vi "passTestNew.vi"(10 "Initial channel":T2) -> (0 "Enum 2":T1)   [LabVIEW 2017]
uses:
  passTestStates.ctl
  <extravilib>/ChannelInstances/Lossy Stream-t'AI Input.ctl'/)Channel.ctl
  Core/AI Input.ctl
  Core/AI Robot.ctl
  Intel/Functions Enum.ctl
  Intel/AttackerStates.ctl
  Core/AI Ball.ctl
  Core/Field Size.ctl
  Core/AI Judge.ctl
  Intel/Command Enum.ctl
  Util/Events/Events.ctl
  <extravilib>/ChannelInstances/Lossy Stream-dbl/Read With Abort.vi
  <extravilib>/ChannelInstances/Lossy Stream-t'AI Input.ctl'/Read With Abort.vi
  <extravilib>/ChannelInstances/Lossy Stream-t'passTestStates.ctl'/Write With Abort.vi
  <extravilib>/ChannelInstances/Lossy Stream-t'passTestStates.ctl'/Read With Abort.vi
  <extravilib>/ChannelInstances/Lossy Stream-dbl/Write With Abort.vi
  <extravilib>/ChannelInstances/Lossy Stream-t'AI Input.ctl'/Write With Abort.vi
  <extravilib>/ChannelInstances/Lossy Stream-dbl/EndpointRead.vi
  <extravilib>/ChannelInstances/Lossy Stream-t'AI Input.ctl'/EndpointRead.vi
  <extravilib>/ChannelInstances/Lossy Stream-t'passTestStates.ctl'/Endpoint.vi
  <extravilib>/ChannelInstances/Lossy Stream-t'passTestStates.ctl'/EndpointRead.vi
  <extravilib>/ChannelInstances/Lossy Stream-dbl/Endpoint.vi
  <extravilib>/ChannelInstances/Lossy Stream-t'AI Input.ctl'/Endpoint.vi
  <extravilib>/ChannelInstances/Lossy Stream-t'AI Input.ctl'/Instantiate.vi
  <extravilib>/ChannelInstances/Lossy Stream-t'AI Input.ctl'/)Channel.vi
  <resource>/ChannelSupport/_ChannelSupport/WaitIfNeeded.vi
  <extravilib>/ChannelInstances/Lossy Stream-t'passTestStates.ctl'/Instantiate.vi
  <extravilib>/ChannelInstances/Lossy Stream-t'passTestStates.ctl'/)Channel.vi
  <extravilib>/ChannelInstances/Lossy Stream-dbl/Instantiate.vi
  <extravilib>/ChannelInstances/Lossy Stream-dbl/)Channel.vi
  <extravilib>/ChannelInstances/Lossy Stream-t'passTestStates.ctl'.lvlib
  <extravilib>/ChannelInstances/Lossy Stream-t'AI Input.ctl'.lvlib
  <extravilib>/ChannelInstances/Lossy Stream-dbl.lvlib
panel:
  out "Enum":T1
  out "ID Kicker Robot":dbl
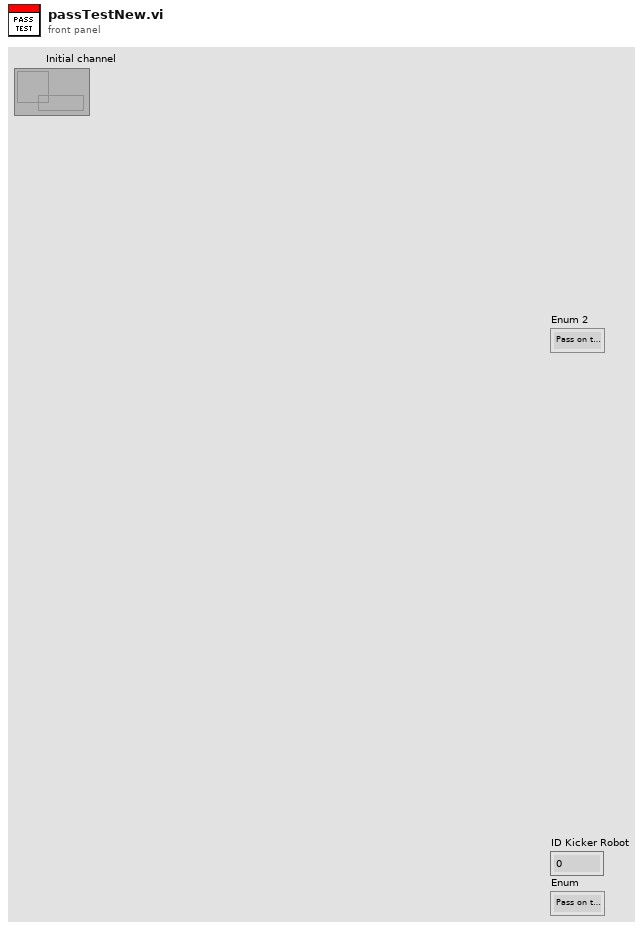
[diagram p1: front panel]
types:
  T1 = typedef "passTestStates.ctl" = enum16{"Pass on the way", "Ball stops", "Pass intercepted", "Ball out of the field", "Ball missed robot", "Need more force to pass", "Too much force", "Correct pass", "Keep ball possesion", "Robot kicked the ball"}
  T2 = typedef "Lossy Stream-t'AI Input.ctl'.lvlib/)Channel.ctl" = refnum<queue>
  T3 = typedef "AI Input.ctl" = cluster{"our_robots":T4[], "enemy_robots":T4[], "balls":T7[], "geometry":T8, "IA Judge":T9, "Received Timestamp":timestamp, "Events":T11}
  T4 = typedef "AI Robot.ctl" = cluster{"id":u32, "function":T5, "x":dbl, "y":dbl, "orientation":dbl, "v_tangent":dbl, "v_normal":dbl, "v_ang":dbl, "kick_x":dbl, "kick_z":dbl, "dribble":bool, "Timestamp":timestamp, "dest_x":dbl, "dest_y":dbl, "dest_orientation":dbl, "estimatives":cluster{"est_v_tangent":dbl, "est_v_normal":dbl, "est_vx":dbl, "est_vy":dbl, "Pos Robot Est":dbl[]}, "dest_x_kick":dbl, "dest_y_kick":dbl, "Gap Coord":dbl[], "States":T6}
  T5 = typedef "Functions Enum.ctl" = enum16{"Attacker", "Goalie", "Defender", "Striker", "Goto 0", "Dummy", "Kicker", "ZigZag"}
  T6 = typedef "AttackerStates.ctl" = enum16{"Pass", "GoToTangent", "BallGetting", "GoToKick", ""}
  T7 = typedef "AI Ball.ctl" = cluster{"x":dbl, "y":dbl, "timestamp":timestamp, "Vel_x":dbl, "Vel_y":dbl, "Pos Bola Est":dbl[]}
  T8 = typedef "Field Size.ctl" = cluster{"line_width":u32, "field_length":u32, "field_width":u32, "boundary_width":u32, "referee_width":u32, "goal_width":u32, "goal_depth":u32, "goal_wall_width":u32, "center_circle_radius":u32, "defense_radius":u32, "defense_stretch":u32, "free_kick_from_defense_dist":u32, "penalty_spot_from_field_line_dist":u32, "penalty_line_from_spot_dist":u32}
  T9 = typedef "AI Judge.ctl" = cluster{"stage":string, "command":string, "our_goalie_id":dbl, "enemy_goalie_id":dbl, "command enum":T10, "Time":enum16{"Azul", "Amarelo"}}
  T10 = typedef "Command Enum.ctl" = enum16{"Halt", "Stop", "Force Start", "PKA Normal Start", "Prepare Kickoff Ally", "PKE Normal Start", "Prepare Kickoff Enemy", "Prepare Penalty Ally", "PPA Normal Start", "Prepare Penalty Enemy", "PPE Normal Start", "Direct Free Enemy", "Direct Free Ally", "Indirect Free Enemy", "Indirect Free Ally", "Timeout Enemy", "Timeout Ally", "Goal Enemy", "Goal Ally", "Ball Placement Enemy", "Ball Placement Ally", "Normal Half Time", "Extra Time Break", "Extra Half Time", "None", "Post Game"}
  T11 = typedef "Events.ctl" = cluster{"Touch":bool, "Ball out":bool, "id touch":dbl, "Ball out of \nVision":bool, "Ball inside \nGoalie area":bool, "Robot not responding":bool, "Robots responding status":dbl[], "Enemy Ball \nPossession":bool, "Pass State":bool, "id end of pass":dbl, "Kick":bool, "Id ini Possession":dbl, "Ball Possesion":bool, "Id Possesion":dbl}
  T12 = typedef "Lossy Stream-t'passTestStates.ctl'.lvlib/)Channel.ctl" = refnum<queue>
  T13 = typedef "Lossy Stream-dbl.lvlib/)Channel.ctl" = refnum<queue>
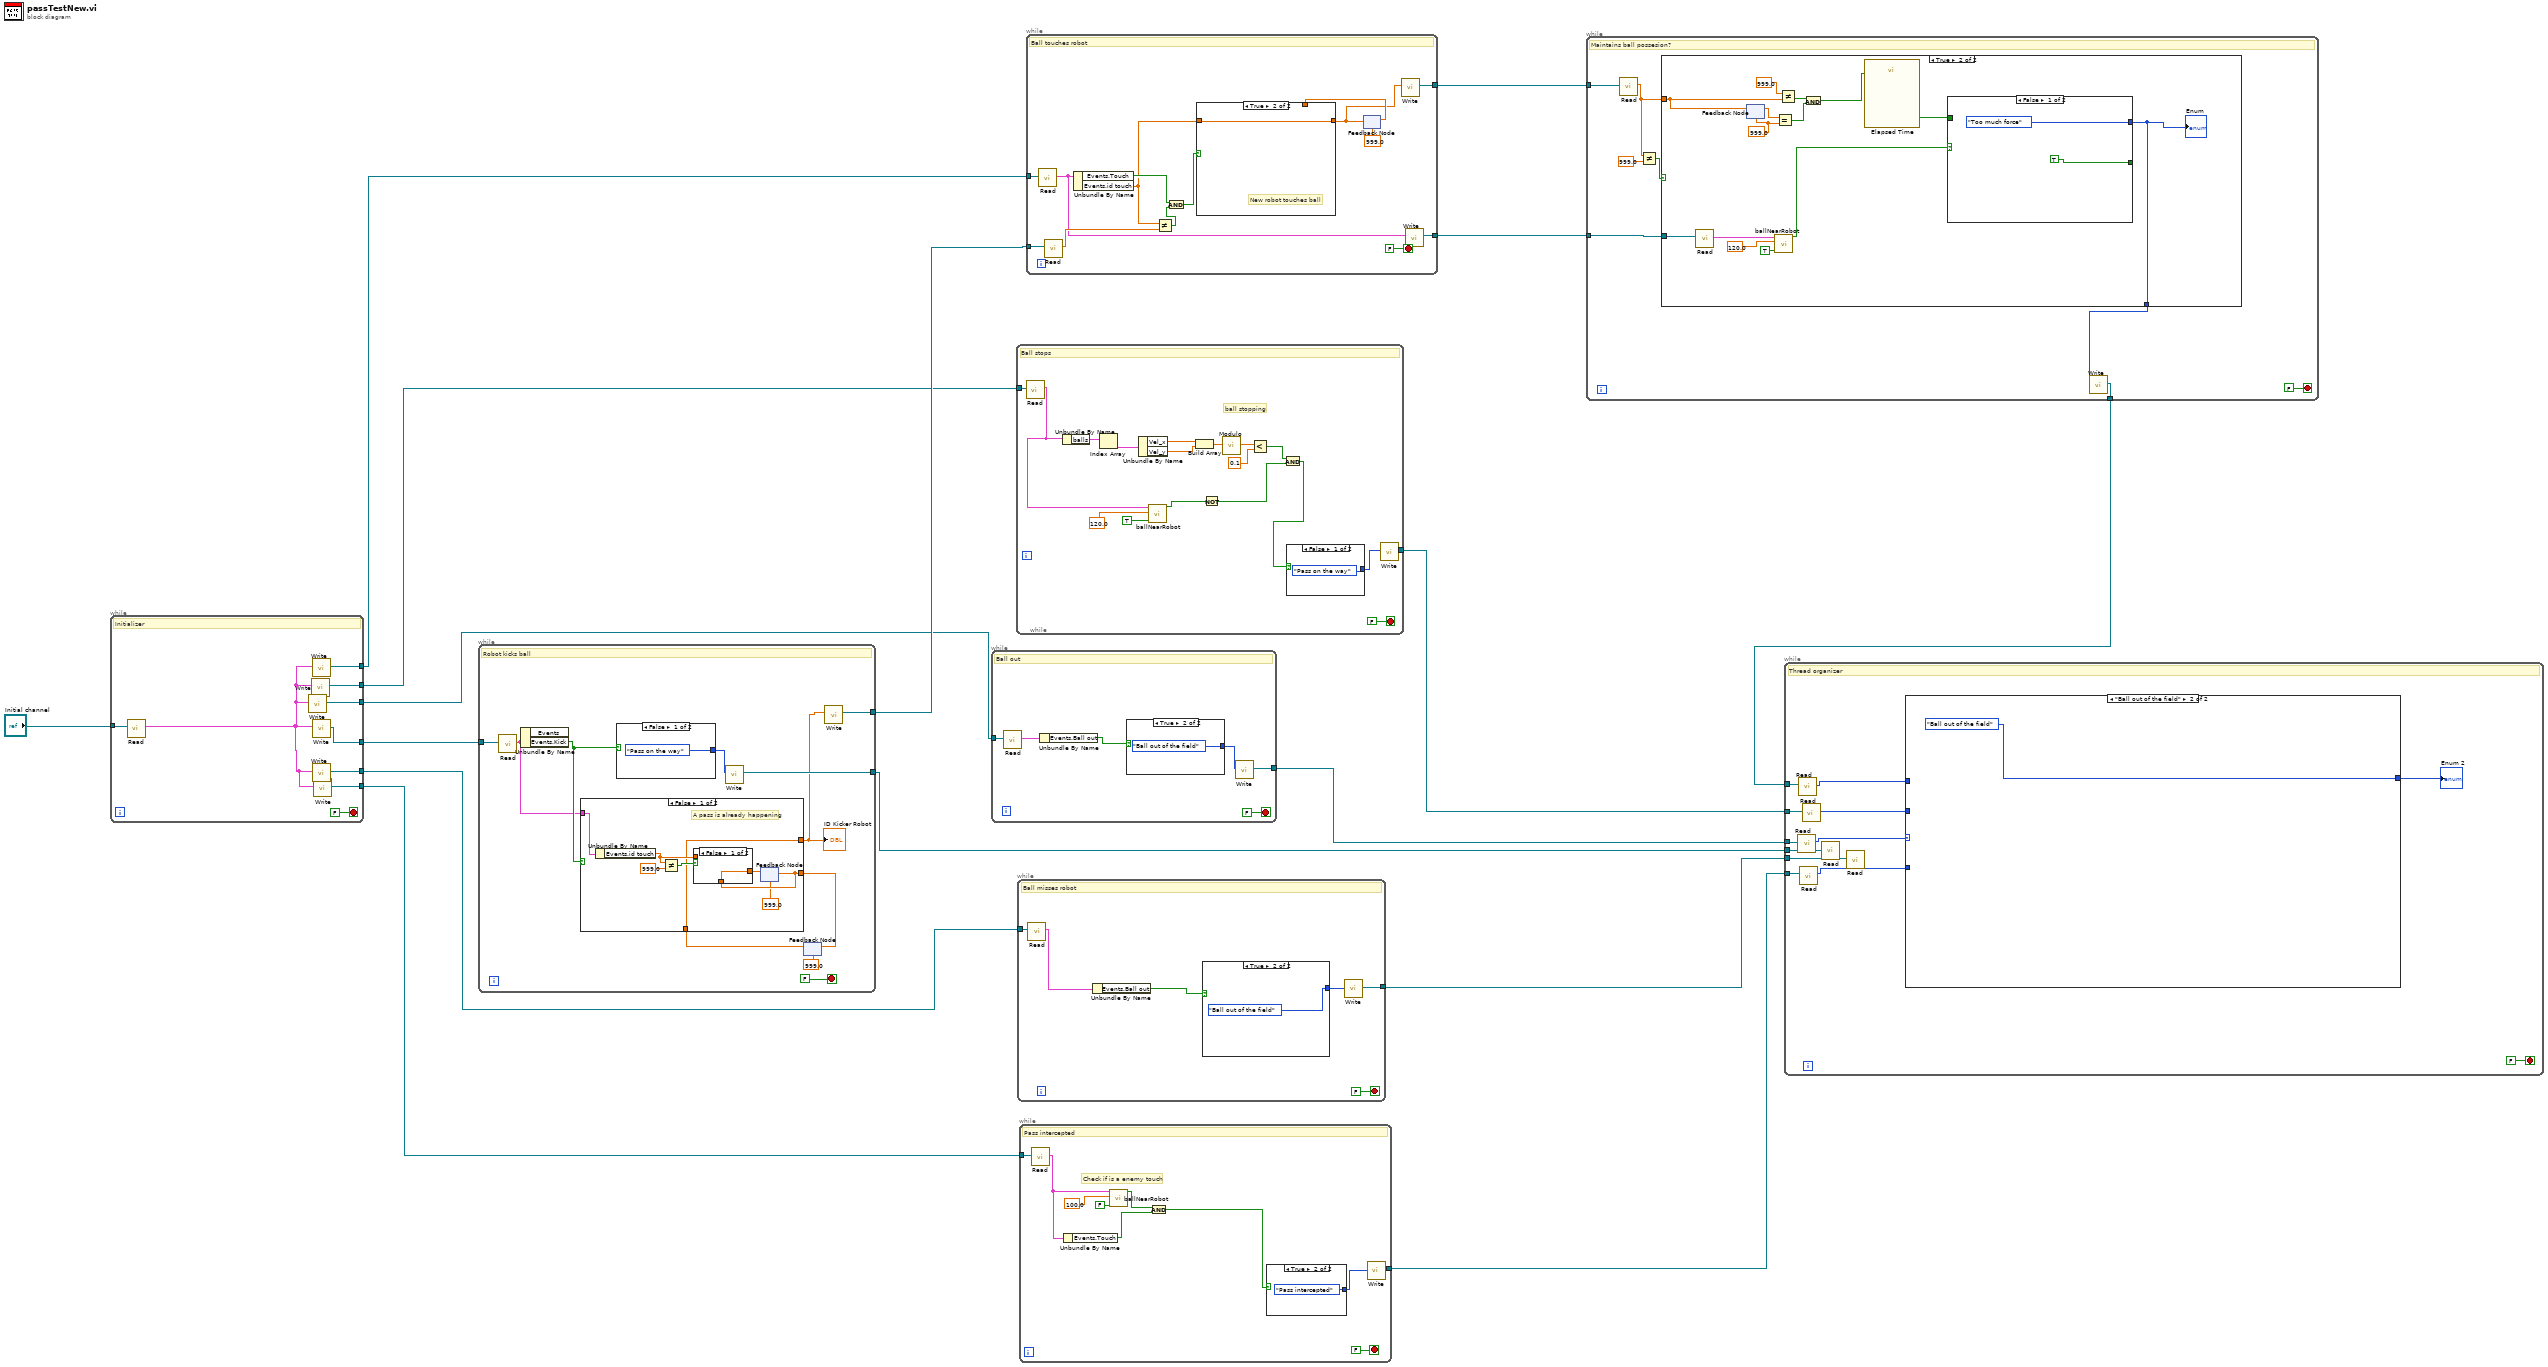
[diagram p0: block diagram]
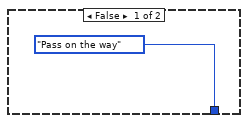
[diagram p2: hidden frame]
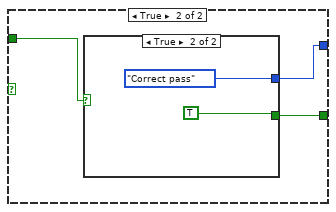
[diagram p3: hidden frame]
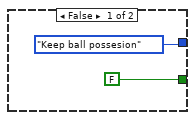
[diagram p4: hidden frame]
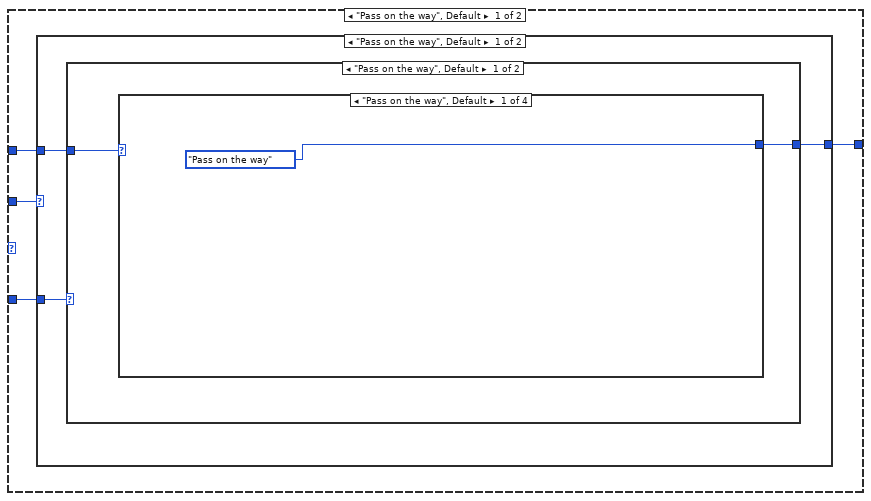
[diagram p5: hidden frame]
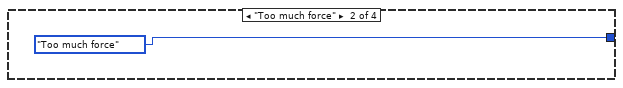
[diagram p6: hidden frame]
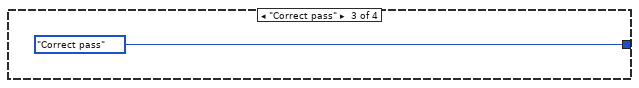
[diagram p7: hidden frame]
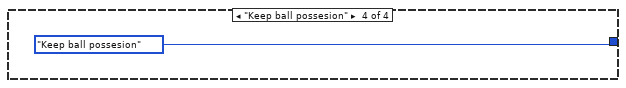
[diagram p8: hidden frame]
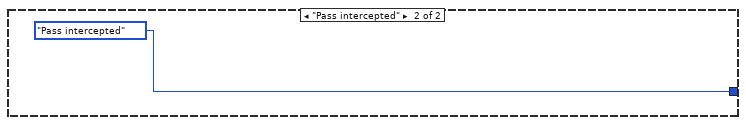
[diagram p9: hidden frame]
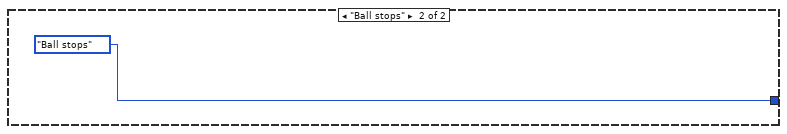
[diagram p10: hidden frame]
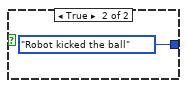
[diagram p14: hidden frame]
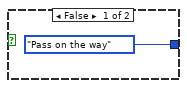
[diagram p15: hidden frame]
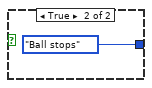
[diagram p16: hidden frame]
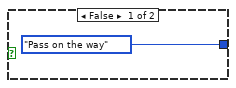
[diagram p17: hidden frame]
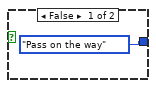
[diagram p18: hidden frame]
diagram:
  n1 = while {
    tunnel: "Initial channel" -> [w25]
    tunnel: [w24] -> w6
    tunnel: [w23] -> w3
    tunnel: [w21] -> w5
    tunnel: [w20] -> w4
    tunnel: [w19] -> w2
    tunnel: [w17] -> w1
    stop <- FALSE stop-if-true
    # "Initializer"
    n2 = call <extravilib>:"Read.vi"("channel"=w25) -> ("element"=w18:T3)  [unwired: 5 in, 5 out]
    n3 = call <extravilib>:"Write.vi"("element"=w18) -> ("channel"=w23:T2)  [unwired: 8 in, 2 out]
    n4 = call <extravilib>:"Write.vi"("element"=w18) -> ("channel"=w19:T2)  [unwired: 8 in, 2 out]
    n5 = call <extravilib>:"Write.vi"("element"=w18) -> ("channel"=w17:T2)  [unwired: 8 in, 2 out]
    n6 = call <extravilib>:"Write.vi"("element"=w18) -> ("channel"=w24:T2)  [unwired: 8 in, 2 out]
    n7 = call <extravilib>:"Write.vi"("element"=w18) -> ("channel"=w20:T2)  [unwired: 8 in, 2 out]
    n8 = call <extravilib>:"Write.vi"("element"=w18) -> ("channel"=w21:T2)  [unwired: 8 in, 2 out]
  }
  n9 = while {
    tunnel: [w35] -> w8
    tunnel: w6 -> [w33]
    tunnel: [w27] -> w16
    stop <- FALSE stop-if-true
    # "Robot kicks ball"
    n10 = call <extravilib>:"Read.vi"("channel"=w33) -> ("element"=w31:T3)  [unwired: 5 in, 5 out]
    n11 = Unbundle By Name(w31) -> ("Events.Kick"=w32:bool)  [unwired: 1 out]
    n12 = case shown="False" w32 {
      tunnel: [passTestStates."Pass on the way" passTestStates."Robot kicked the ball"] -> w34
      frame False {
      }
      frame True {
      }
    }
    n13 = call <extravilib>:"Write.vi"("element"=w34) -> ("channel"=w35:T12)  [unwired: 8 in, 2 out]
    n14 = feedback #1(999.0 ("id touch")) -> (w29:dbl)
    n15 = case shown="False" w32 {
      tunnel: w31 -> [w44 _]
      tunnel: [w39 w47] -> w30
      tunnel: w29 -> [w37 w47]
      tunnel: [w37 w47] -> w28
      frame False {
        # "A pass is already happening"
        n16 = Unbundle By Name(w44) -> ("Events.id touch"=w41:dbl)
        n17 = Not Equal?(x=w41, y=999.0) -> (x != y?=w42:bool)
        n18 = feedback #2(999.0 ("id touch")) -> (w39:dbl)
        n19 = case shown="False" w42 {
          tunnel: w41 -> [_ w46]
          tunnel: [w45 w46] -> w40
          tunnel: w39 -> [w45 _]
          frame False {
          }
          frame True {
          }
        }
        n20 = feedback-in #2(w40) -> ()
      }
      frame True {
        # "A new pass is starting"
      }
    }
    "ID Kicker Robot" <- w28
    n21 = feedback-in #1(w30) -> ()
    n22 = call <extravilib>:"Write.vi"("element"=w28) -> ("channel"=w27:T13)  [unwired: 8 in, 2 out]
  }
  n23 = while {
    tunnel: [w54] -> w11
    tunnel: w3 -> [w51]
    stop <- FALSE stop-if-true
    # "Ball out"
    n24 = call <extravilib>:"Read.vi"("channel"=w51) -> ("element"=w50:T3)  [unwired: 5 in, 5 out]
    n25 = Unbundle By Name(w50) -> ("Events.Ball out"=w53:bool)
    n26 = case shown="True" w53 {
      tunnel: [passTestStates."Pass on the way" passTestStates."Ball out of the field"] -> w52
      frame False {
      }
      frame True {
      }
    }
    n27 = call <extravilib>:"Write.vi"("element"=w52) -> ("channel"=w54:T12)  [unwired: 8 in, 2 out]
  }
  n28 = while {
    tunnel: w2 -> [w60]
    tunnel: [w58] -> w10
    stop <- FALSE stop-if-true
    # "ball stopping"
    # "Ball stops"
    n29 = call <extravilib>:"Read.vi"("channel"=w60) -> ("element"=w59:T3)  [unwired: 5 in, 5 out]
    n30 = Unbundle By Name(w59) -> ("balls"=w75:T7[])
    n31 = Index Array(array=w75) -> (element=w74:T7)  [unwired: 1 in]
    n32 = Unbundle By Name(w74) -> ("Vel_x"=w73:dbl, "Vel_y"=w72:dbl)
    n33 = call "ballNearRobot.vi"("Our robots?"=TRUE, "Distance"=120.0, "IA state"=w59) -> ("Near to some robot"=w67:bool)  [unwired: 7 in, 1 out]
    n34 = Build Array(w73, w72) -> (w71:dbl[])
    n35 = Not(x=w67) -> (.not. x?=w64:bool)
    n36 = call "Modulo.vi"("2D vector"=w71) -> ("Modulo"=w70:dbl)  [unwired: 10 in]
    n37 = Less?(x=w70, y=0.1) -> (x < y?=w68:bool)
    n38 = And(x=w68, y=w64) -> (x .and. y?=w61:bool)
    n39 = case shown="False" w61 {
      tunnel: [passTestStates."Pass on the way" passTestStates."Ball stops"] -> w62
      frame False {
      }
      frame True {
      }
    }
    n40 = call <extravilib>:"Write.vi"("element"=w62) -> ("channel"=w58:T12)  [unwired: 8 in, 2 out]
  }
  n41 = while {
    tunnel: [w81] -> w12
    tunnel: w4 -> [w80]
    stop <- FALSE stop-if-true
    # "Ball misses robot"
    n42 = call <extravilib>:"Read.vi"("channel"=w80) -> ("element"=w79:T3)  [unwired: 5 in, 5 out]
    n43 = Unbundle By Name(w79) -> ("Events.Ball out"=w78:bool)
    n44 = case shown="True" w78 {
      tunnel: [passTestStates."Pass on the way" passTestStates."Ball out of the field"] -> w82
      frame False {
      }
      frame True {
      }
    }
    n45 = call <extravilib>:"Write.vi"("element"=w82) -> ("channel"=w81:T12)  [unwired: 8 in, 2 out]
  }
  n46 = while {
    tunnel: w5 -> [w91]
    tunnel: [w86] -> w13
    stop <- FALSE stop-if-true
    # "Check if is a enemy touch"
    # "Pass intercepted"
    n47 = call <extravilib>:"Read.vi"("channel"=w91) -> ("element"=w90:T3)  [unwired: 5 in, 5 out]
    n48 = Unbundle By Name(w90) -> ("Events.Touch"=w89:bool)
    n49 = call "ballNearRobot.vi"("Our robots?"=FALSE, "Distance"=100.0, "IA state"=w90) -> ("Near to some robot"=w93:bool)  [unwired: 7 in, 1 out]
    n50 = And(x=w93, y=w89) -> (x .and. y?=w88:bool)
    n51 = case shown="True" w88 {
      tunnel: [passTestStates."Pass on the way" passTestStates."Pass intercepted"] -> w87
      frame False {
      }
      frame True {
      }
    }
    n52 = call <extravilib>:"Write.vi"("element"=w87) -> ("channel"=w86:T12)  [unwired: 8 in, 2 out]
  }
  n53 = while {
    tunnel: w1 -> [w110]
    tunnel: w16 -> [w108]
    tunnel: [w100] -> w15
    tunnel: [w98] -> w14
    stop <- FALSE stop-if-true
    # "Ball touches robot"
    n54 = call <extravilib>:"Read.vi"("channel"=w110) -> ("element"=w99:T3)  [unwired: 5 in, 5 out]
    n55 = call <extravilib>:"Read.vi"("channel"=w108) -> ("element"=w107:dbl)  [unwired: 5 in, 5 out]
    n56 = Unbundle By Name(w99) -> ("Events.Touch"=w106:bool, "Events.id touch"=w103:dbl)
    n57 = Not Equal?(x=w103, y=w107) -> (x != y?=w105:bool)
    n58 = And(x=w106, y=w105) -> (x .and. y?=w104:bool)
    n59 = feedback #3(999.0 ("id touch")) -> (w102:dbl)
    n60 = case shown="True" w104 {
      tunnel: w103 -> [_ w113]
      tunnel: [w112 w113] -> w101
      tunnel: w102 -> [w112 _]
      frame False {
      }
      frame True {
        # "New robot touches ball"
      }
    }
    n61 = feedback-in #3(w101) -> ()
    n62 = call <extravilib>:"Write.vi"("element"=w101) -> ("channel"=w100:T13)  [unwired: 8 in, 2 out]
    n63 = call <extravilib>:"Write.vi"("element"=w99) -> ("channel"=w98:T2)  [unwired: 8 in, 2 out]
  }
  n64 = while {
    tunnel: w15 -> [w117]
    tunnel: w14 -> [w120]
    tunnel: [w118] -> w9
    stop <- FALSE stop-if-true
    # "Maintains ball possesion?"
    n65 = call <extravilib>:"Read.vi"("channel"=w117) -> ("element"=w115:dbl)  [unwired: 5 in, 5 out]
    n66 = Not Equal?(x=w115, y=999.0) -> (x != y?=w114:bool)
    n67 = case shown="True" w114 {
      tunnel: w120 -> [_ w134]
      tunnel: [passTestStates."Pass on the way" w124] -> w119
      tunnel: w115 -> [_ w123]
      frame False {
      }
      frame True {
        w131 = 999.0 ("element")
        n68 = call <extravilib>:"Read.vi"("channel"=w134) -> ("element"=w133:T3)  [unwired: 5 in, 5 out]
        n69 = feedback #4(w131) -> (w130:dbl)
        n70 = feedback-in #4(w123) -> ()
        n71 = call "ballNearRobot.vi"("Our robots?"=TRUE, "Distance"=120.0, "IA state"=w133) -> ("Near to some robot"=w132:bool)  [unwired: 7 in, 1 out]
        n72 = Equal?(x=w130, y=w131) -> (x = y?=w129:bool)
        n73 = Not Equal?(x=999.0 ("element"), y=w123) -> (x != y?=w128:bool)
        n74 = And(x=w128, y=w129) -> (x .and. y?=w126:bool)
        n75 = call "Elapsed Time"("Reset"=w126) -> ("Time has Elapsed"=w125:bool)  [unwired: 11 in, 7 out]
        n76 = case shown="False" w132 {
          tunnel: [passTestStates."Too much force" w141] -> w124
          tunnel: [TRUE ("y") w140] -> _
          tunnel: w125 -> [_ w139]
          frame False {
          }
          frame True {
            n77 = case shown="True" w139 {
              tunnel: [passTestStates."Keep ball possesion" passTestStates."Correct pass"] -> w141
              tunnel: [FALSE ("y") TRUE ("y")] -> w140
              frame False {
              }
              frame True {
              }
            }
          }
        }
        "Enum" <- w124
      }
    }
    n78 = call <extravilib>:"Write.vi"("element"=w119) -> ("channel"=w118:T12)  [unwired: 8 in, 2 out]
  }
  n79 = while {
    tunnel: w13 -> [w151]
    tunnel: w12 -> [w152]
    tunnel: w11 -> [w154]
    tunnel: w10 -> [w155]
    tunnel: w9 -> [w156]
    tunnel: w8 -> [w153]
    stop <- FALSE stop-if-true
    # "Thread organizer"
    n80 = call <extravilib>:"Read.vi"("channel"=w154) -> ("element"=w150:T1)  [unwired: 5 in, 5 out]
    n81 = call <extravilib>:"Read.vi"("channel"=w156) -> ("element"=w147:T1)  [unwired: 5 in, 5 out]
    n82 = call <extravilib>:"Read.vi"("channel"=w151) -> ("element"=w148:T1)  [unwired: 5 in, 5 out]
    n83 = call <extravilib>:"Read.vi"("channel"=w155) -> ("element"=w149:T1)  [unwired: 5 in, 5 out]
    n84 = call <extravilib>:"Read.vi"("channel"=w153) -> ()  [unwired: 5 in, 6 out]
    n85 = call <extravilib>:"Read.vi"("channel"=w152) -> ()  [unwired: 5 in, 6 out]
    n86 = case shown="\"Ball out of the field\"" w150 {
      tunnel: w149 -> [w161 _]
      tunnel: w148 -> [w160 _]
      tunnel: w147 -> [w159 _]
      tunnel: [w158 passTestStates."Ball out of the field"] -> w146
      frame "Pass on the way", Default {
        n87 = case shown="\"Pass on the way\", Default" w161 {
          tunnel: w160 -> [w164 _]
          tunnel: w159 -> [w163 _]
          tunnel: [w162 passTestStates."Ball stops"] -> w158
          frame "Pass on the way", Default {
            n88 = case shown="\"Pass on the way\", Default" w164 {
              tunnel: w163 -> [w166 _]
              tunnel: [w165 passTestStates."Pass intercepted"] -> w162
              frame "Pass on the way", Default {
                n89 = case shown="\"Pass on the way\", Default" w166 {
                  tunnel: [passTestStates."Pass on the way" passTestStates."Too much force" passTestStates."Correct pass" passTestStates."Keep ball possesion"] -> w165
                  frame "Pass on the way", Default {
                  }
                  frame "Too much force" {
                  }
                  frame "Correct pass" {
                  }
                  frame "Keep ball possesion" {
                  }
                }
              }
              frame "Pass intercepted" {
              }
            }
          }
          frame "Ball stops" {
          }
        }
      }
      frame "Ball out of the field" {
      }
    }
    "Enum 2" <- w146
  }
